vi "RSZVB Get Time Out.vi"(8 "error in (no error)":errorcluster {"code" format="%.0x"}, 11 "VISA session":refnum<visa-resource-name>) -> (0 "error out":errorcluster {"code" format="%.0x"}, 1 "Timeout":i32, 3 "dup VISA session":refnum<visa-resource-name>)   [LabVIEW 2011]
doc: "Returns the timeout value for driver I/O transactions in milliseconds.\n\nThe timeout period may vary on computer platforms."
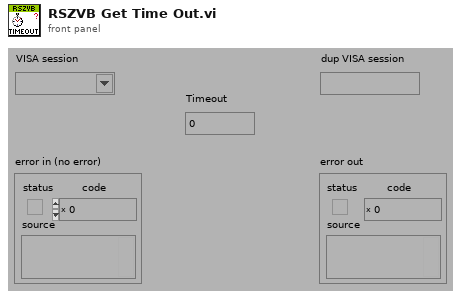
[diagram p1: front panel]
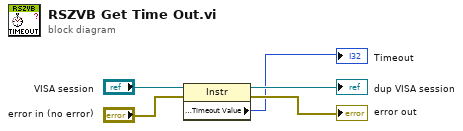
[diagram p0: block diagram]
diagram:
  n1 = property class="Instr"(reference="VISA session", error in="error in (no error)") -> (reference out=→"dup VISA session":refnum<visa-resource-name>, error out=→"error out":errorcluster, "General Settings:Timeout Value"=→"Timeout":u32)
